vi "Encode.vi"(9 "word count":u8, 10 "param config":T1[](array[typedef]), 11 "parameters in":dbl[](array[numeric])) -> (3 "words out":u16[](array[numeric]))   [LabVIEW 2020]
uses:
  _typedefs/parameter_config_encoding_type.ctl
  _typedefs/parameter_config_type_type.ctl
  _typedefs/parameter_config_type.ctl
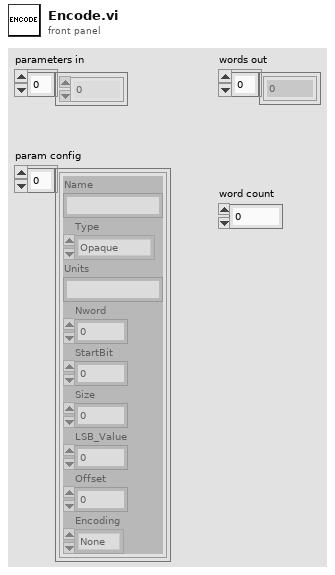
[diagram p1: front panel]
types:
  T1 = typedef "parameter_config_type.ctl" = cluster{"Name":string, "Type":T2, "Units":string, "Nword":i32, "StartBit":i32, "Size":i32, "LSB_Value":i32, "Offset":i32, "Encoding":T3}
  T2 = typedef "parameter_config_type_type.ctl" = enum16{"Opaque", "Enum", "Float", "Integer", "Bcd", "Bool"}
  T3 = typedef "parameter_config_encoding_type.ctl" = enum16{"None", "2-complement", "Unsigned"}
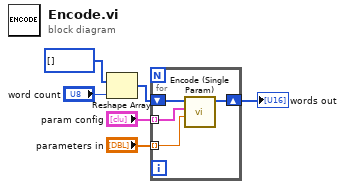
[diagram p0: block diagram]
diagram:
  n1 = Reshape Array(u16[] [] ("words out"), "word count") -> (w2:u16[])
  n2 = for {
    tunnel: "param config" -> [w10] mode=indexing
    tunnel: "parameters in" -> [w7] mode=indexing
    shift-right: [w9] -> w1
    shift-left: w2 -> [w8]
    n3 = call "Encode (Single Param).vi"("parameter in"=w7, "parameter configuration"=w10, "words in"=w8) -> ("words out"=w9:u16[])  [unwired: 8 in]
  }
  "words out" <- w1
